vi "tm_startcapture_b.vi"(8 "error in (no error)":errorcluster {"code" format="%.0x"}, 11 "Handle in":u32) -> (0 "error out":errorcluster {"code" format="%.0x"}, 3 "Handle out":u32)   [LabVIEW 2015]
uses:
  tmcamcon.dll
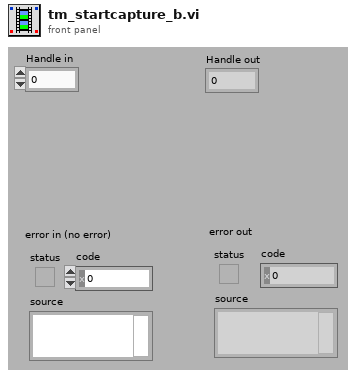
[diagram p1: front panel]
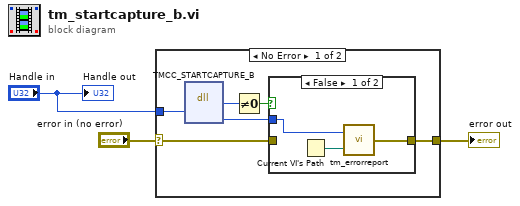
[diagram p0: block diagram]
diagram:
  n1 = case shown="No Error" "error in (no error)" {
    selector: "error in (no error)" -> [w4 w14]
    tunnel: [w7 w14] -> w1
    tunnel: "Handle in" -> [w8 _]
    frame No Error {
      n2 = dll-call lib="tmcamcon.dll" fn="TMCC_STARTCAPTURE_B"("index"=w8) -> ("return type"=w9:u32, "Erval"=w6:i32)  [unwired: 5 in, 2 out]
      n3 = Not Equal To 0?(x=w9) -> (x != 0?=w5:bool)
      n4 = case shown="False" w5 {
        tunnel: w4 -> [_ w13]
        tunnel: [w11 w13] -> w7
        tunnel: w6 -> [w10 _]
        frame False {
          n5 = Current VI's Path() -> (path=w12:path)
          n6 = call "tm_errorreport.vi"("Source"=w12, "Error"=w10) -> ("error out"=w11:errorcluster)
        }
        frame True {
        }
      }
    }
    frame Error {
    }
  }
  "error out" <- w1
  "Handle out" <- "Handle in"
